vi "Dashboard globals.vi"() -> ()   [LabVIEW 2018]
panel:
  in  "Right y":sgl
  in  "Left y":sgl
  in  "Right x":sgl
  in  "Left x":sgl
  in  "Right width":sgl
  in  "Left width":sgl
  in  "Right height":sgl
  in  "Left height":sgl
  out "Desired Target":T1(radio)=enum."Rocket or Loading Station"
  in  "Enable Vision\nProcessing":bool
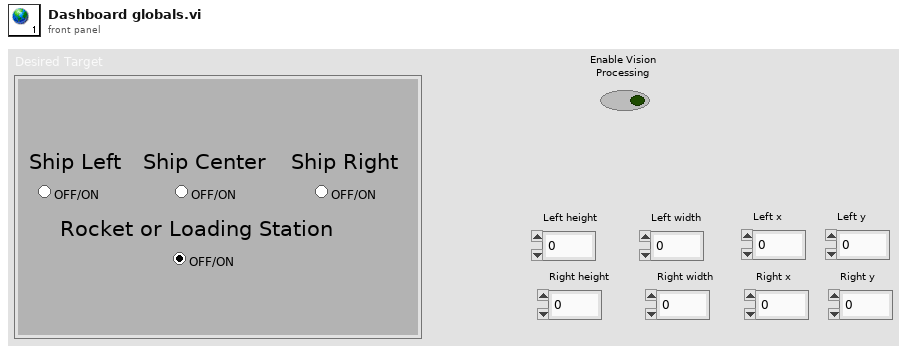
[diagram p1: front panel]
types:
  T1 = enum32{"Ship Left", "Ship Center", "Ship Right", "Rocket or Loading Station"}
diagram:
